vi "JL_RelayVerification_WaitforRelayState.vi"(0 "Expected Electric Loads":T1, 1 "Min Execution Time":dbl, 2 "Timeout":dbl, 5 "Care Electric Loads":T1={"Steam Relay"=TRUE, "Drum Motor"=TRUE, "Drum Direction"=TRUE, "Heater 1 / Bottom"=TRUE, "Heater 2 / Top"=TRUE, "Drum Light"=TRUE}, 11 "Error In":errorcluster) -> (4 "Pass/Fail?":bool, 6 "Report Text":string, 8 "Execution Time":dbl, 15 "Error Out":errorcluster)   [LabVIEW 2016]
uses:
  Type Defs/JL_ElectricRelay_Loads.ctl
  <vilib>/DAQmx/read.llb/DAQmx Read (Digital 1D Bool NChan 1Samp 1Line).vi
  <vilib>/DAQmx/create/channels.llb/DAQmx Create Channel (DI-Digital Input).vi
  <vilib>/DAQmx/miscellaneous.llb/DAQmx Fill In Error Info.vi
panel:
  in  "DAQ Lines":tag="9401_1/port0/line0:7"
  in  "Tab Control":enum32{"Electric"}(tab)
  in  "Stop Button":bool
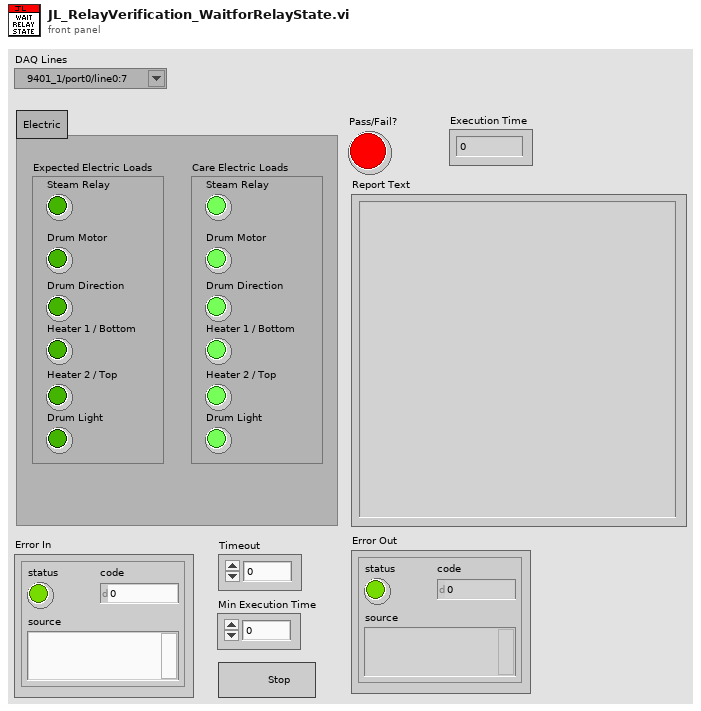
[diagram p1: front panel]
types:
  T1 = typedef "JL_ElectricRelay_Loads.ctl" = cluster{"Steam Relay":bool, "Drum Motor":bool, "Drum Direction":bool, "Heater 1 / Bottom":bool, "Heater 2 / Top":bool, "Drum Light":bool}
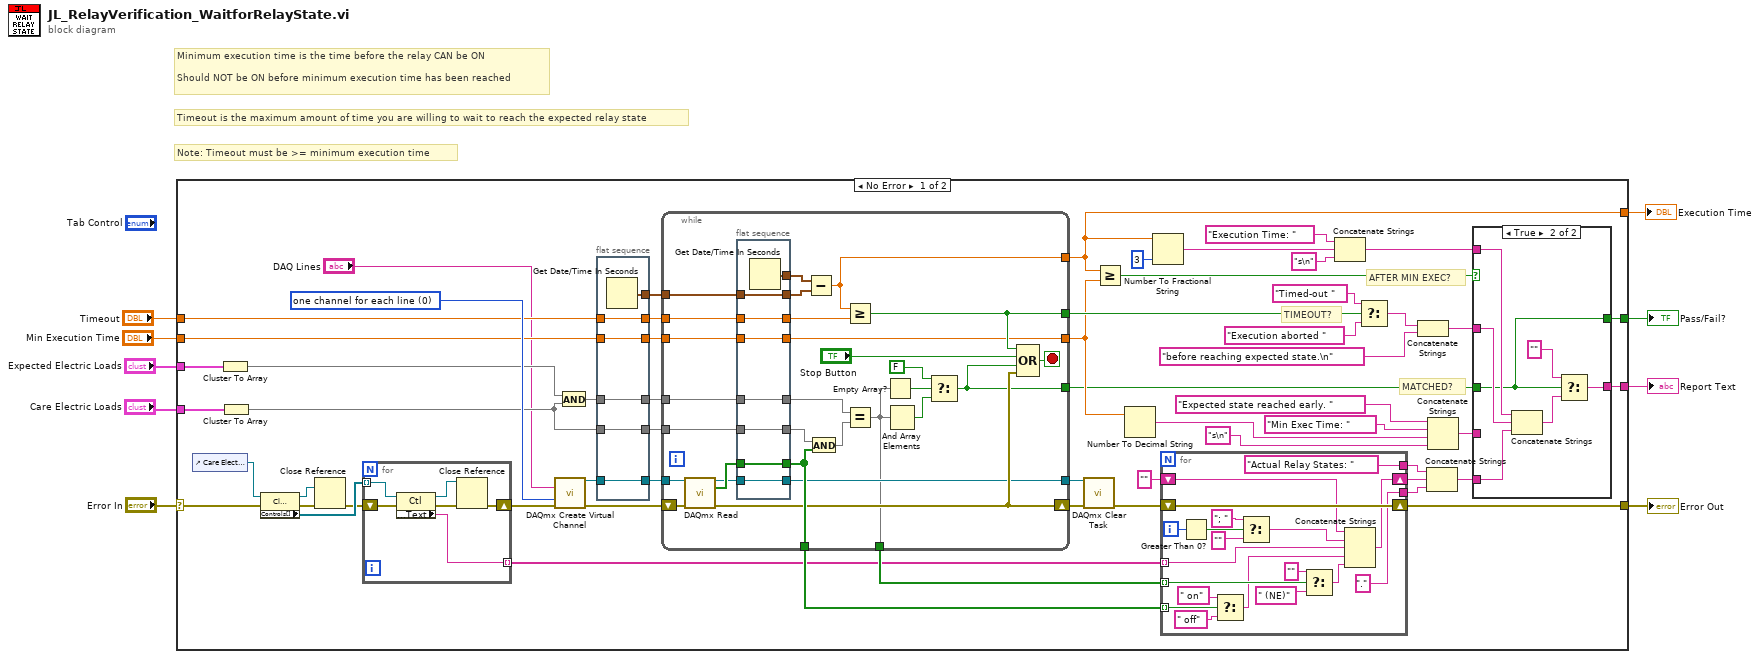
[diagram p0: block diagram]
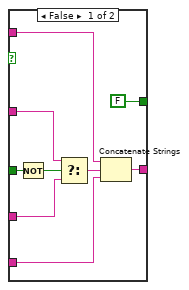
[diagram p2: hidden frame]
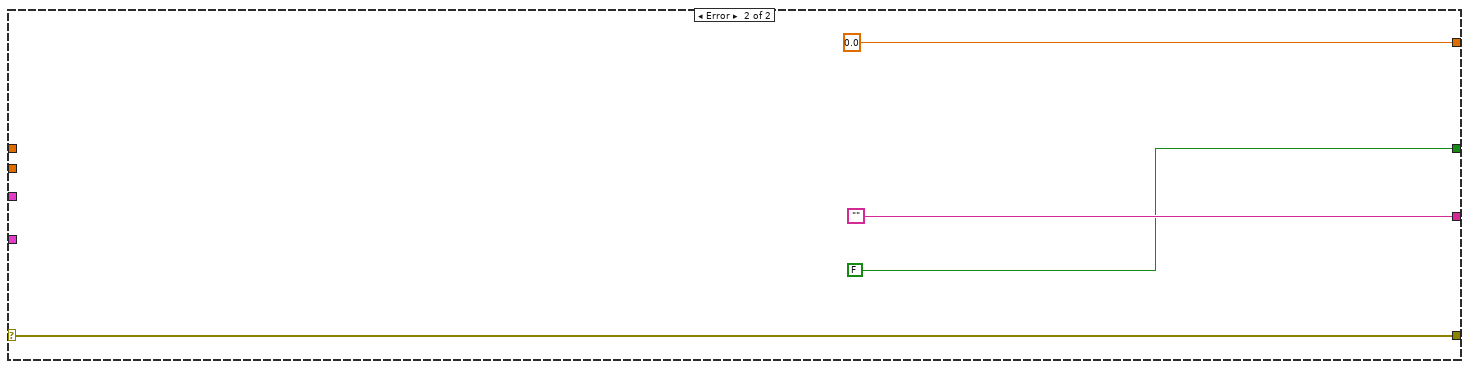
[diagram p3: hidden frame]
diagram:
  # "Note: Timeout must be >= minimum execution time"
  # "Timeout is the maximum amount of time you are willing to wait to reach the expected relay state"
  # "Minimum execution time is the time before the relay CAN be ON\n\nShould NOT be ON before minimum execution time has been reached"
  n1 = case shown="No Error" "Error In" {
    selector: "Error In" -> [w11 w151]
    tunnel: [w43 w151] -> w3
    tunnel: "Timeout" -> [w28 _]
    tunnel: [w31 0.0] -> w7
    tunnel: [w24 FALSE] -> w6
    tunnel: [w29 ""] -> w5
    tunnel: "Min Execution Time" -> [w53 _]
    tunnel: "Expected Electric Loads" -> [w66 _]
    tunnel: "Care Electric Loads" -> [w64 _]
    frame No Error {
      w65 = 0 items=["one channel for each line", "one channel for all lines"] ("line grouping")
      # "TIMEOUT?"
      # "AFTER MIN EXEC?"
      # "MATCHED?"
      n2 = control-ref of="Care Electric Loads"() -> (w12:refnum<vi>)
      n3 = Cluster To Array(cluster=w66) -> (array=w13:bool[])
      n4 = Cluster To Array(cluster=w64) -> (array=w14:bool[])
      n5 = property class="Clust (strict)"(reference=w12, error in=w11) -> (reference out=w18:refnum<vi>, error out=w17:errorcluster, "Controls[]"=w20:refnum<vi>[])
      n6 = Close Reference(reference=w18, error in (no error)=w17) -> (error out=w19:errorcluster)
      n7 = for {
        tunnel: [w73] -> w16 mode=indexing
        tunnel: w20 -> [w71] mode=indexing
        shift-right: [w69] -> w15
        shift-left: w19 -> [w72]
        n8 = property class="Ctl"(reference=w71, error in=w72) -> (reference out=w68:refnum<vi>, error out=w70:errorcluster, "Label.Text"=w73:string)
        n9 = Close Reference(reference=w68, error in (no error)=w70) -> (error out=w69:errorcluster)
      }
      n10 = call-poly <vilib>:"DAQmx Create Virtual Channel.vi"("lines"="DAQ Lines", "line grouping"=w65, "error in"=w15) -> ("task out"=w63:refnum<k21>, "error out"=w37:errorcluster)  [unwired: 11 in]
      n11 = And(x=w13, y=w14) -> (x .and. y?=w54:bool[])
      n12 = flat-sequence {
        tunnel: [w148] -> w55
        tunnel: w63 -> [w149]
        tunnel: [w147] -> w56
        tunnel: [w150] -> w57
        tunnel: w14 -> [w150]
        tunnel: [w149] -> w58
        tunnel: w54 -> [w147]
        tunnel: w53 -> [w146]
        tunnel: [w146] -> w52
        tunnel: w28 -> [w145]
        tunnel: [w145] -> w27
        frame #0 {
          n13 = Get Date/Time In Seconds() -> (seconds since 1Jan1904=w148:timestamp)
        }
      }
      n14 = while {
        tunnel: w55 -> [w126]
        tunnel: w56 -> [w128]
        tunnel: w57 -> [w130]
        tunnel: w58 -> [w136]
        tunnel: [w134] -> w49
        tunnel: [w114] -> w59
        shift-right: [w120] -> w60
        shift-left: w37 -> [w135]
        tunnel: [w113] -> w47
        tunnel: [w109] -> w21
        tunnel: w52 -> [w124]
        tunnel: [w123] -> w30
        tunnel: [w118] -> w31
        tunnel: [w121] -> w46
        tunnel: w27 -> [w117]
        stop <- w133 stop-if-true
        n15 = call-poly <vilib>:"DAQmx Read.vi"("task/channels in"=w136, "error in"=w135) -> ("task out"=w115:refnum<k21>, "data"=w131:bool[], "error out"=w120:errorcluster)  [unwired: 11 in]
        n16 = flat-sequence {
          tunnel: [w144] -> w132
          tunnel: w131 -> [w143]
          tunnel: [w143] -> w121
          tunnel: w130 -> [w142]
          tunnel: [w142] -> w129
          tunnel: w128 -> [w141]
          tunnel: [w141] -> w127
          tunnel: w126 -> [w140]
          tunnel: [w140] -> w125
          tunnel: w124 -> [w139]
          tunnel: [w139] -> w123
          tunnel: w117 -> [w138]
          tunnel: [w138] -> w116
          tunnel: [w137] -> w114
          tunnel: w115 -> [w137]
          frame #0 {
            n17 = Get Date/Time In Seconds() -> (seconds since 1Jan1904=w144:timestamp)
          }
        }
        n18 = Subtract(x=w132, y=w125) -> (x-y=w118:dbl)
        n19 = And(x=w129, y=w121) -> (x .and. y?=w122:bool[])
        n20 = Greater Or Equal?(x=w118, y=w116) -> (x >= y?=w134:bool)
        n21 = Equal?(x=w127, y=w122) -> (x = y?=w113:bool[])
        n22 = Empty Array?(array=w113) -> (empty?=w112:bool)
        n23 = And Array Elements(Boolean array=w113) -> (logical AND=w111:bool)
        n24 = Select(t=FALSE, s=w112, f=w111) -> (s? t:f=w109:bool)
        n25 = Compound Arithmetic op=OR(w134, "Stop Button", w109, w120) -> (w133:bool)
      }
      n26 = call <vilib>:"DAQmx Clear Task.vi"("task in"=w59, "error in"=w60) -> ("error out"=w42:errorcluster)  [unwired: 13 in]
      n27 = Greater Or Equal?(x=w31, y=w30) -> (x >= y?=w25:bool)
      n28 = Number To Decimal String(number=w30) -> (decimal integer string=w44:string)  [unwired: 1 in]
      n29 = Number To Fractional String(number=w31, precision (6)=i16 3) -> (F-format string=w62:string)  [unwired: 2 in]
      n30 = for {
        tunnel: w47 -> [w101] mode=indexing
        shift-right: [w106] -> w40
        shift-left: "" -> [w107]
        shift-right: [w108] -> w43
        shift-left: w42 -> [w108]
        tunnel: w46 -> [w105] mode=indexing
        tunnel: w16 -> [w98] mode=indexing
        tunnel: ["Actual Relay States: " ("string")] -> w39
        tunnel: ["." ("string")] -> w38
        i -> [w97]
        n31 = Greater Than 0?(x=w97) -> (x > 0?=w100:bool)
        n32 = Select(t=" on" ("string"), s=w105, f=" off" ("string")) -> (s? t:f=w93:string)
        n33 = Select(t="; " ("string"), s=w100, f="" ("string")) -> (s? t:f=w95:string)
        n34 = Select(t="" ("string"), s=w101, f=" (NE)" ("string")) -> (s? t:f=w94:string)
        n35 = Concatenate Strings(w107, w95, w98, w93, w94) -> (w106:string)
      }
      n36 = Concatenate Strings("Execution Time: " ("string"), w62, "s\n" ("string")) -> (w26:string)
      n37 = Select(t="Timed-out ", s=w49, f="Execution aborted ") -> (s? t:f=w33:string)
      n38 = Concatenate Strings(w33, "before reaching expected state.\n") -> (w23:string)
      n39 = Concatenate Strings(w39, w40, w38) -> (w36:string)
      n40 = Concatenate Strings("Expected state reached early. " ("string"), "Min Exec Time: " ("string"), w44, "s\n" ("string")) -> (w22:string)
      n41 = case shown="True" w25 {
        tunnel: w36 -> [w82 w89]
        tunnel: [w81 w86] -> w29
        tunnel: w26 -> [w80 w88]
        tunnel: w21 -> [w75 w83]
        tunnel: [FALSE w83] -> w24
        tunnel: w23 -> [w77 w87]
        tunnel: w22 -> [w76 _]
        frame False {
          n42 = Not(x=w75) -> (.not. x?=w74:bool)
          n43 = Select(t=w77, s=w74, f=w76) -> (s? t:f=w78:string)
          n44 = Concatenate Strings(w80, w78, w82) -> (w81:string)
        }
        frame True {
          n45 = Concatenate Strings(w88, w87, w89) -> (w84:string)
          n46 = Select(t="", s=w83, f=w84) -> (s? t:f=w86:string)
        }
      }
    }
    frame Error {
    }
  }
  "Execution Time" <- w7
  "Pass/Fail?" <- w6
  "Report Text" <- w5
  "Error Out" <- w3
